vi "Write.vi"(8 "error in (no error)":errorcluster, 10 "write buffer":string, 11 "uCAN in":refnum<class "uCAN.lvclass">) -> (0 "error out":errorcluster)   [LabVIEW 2021, in "uCanDriver.lvlib" / "uCAN.lvclass"]
doc: "Writes given text on COM port"
uses:
  uCAN.lvclass
  uCAN.lvclass/uCAN.ctl
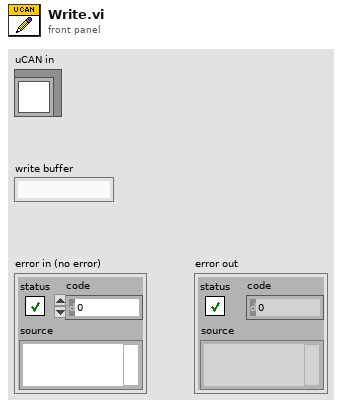
[diagram p1: front panel]
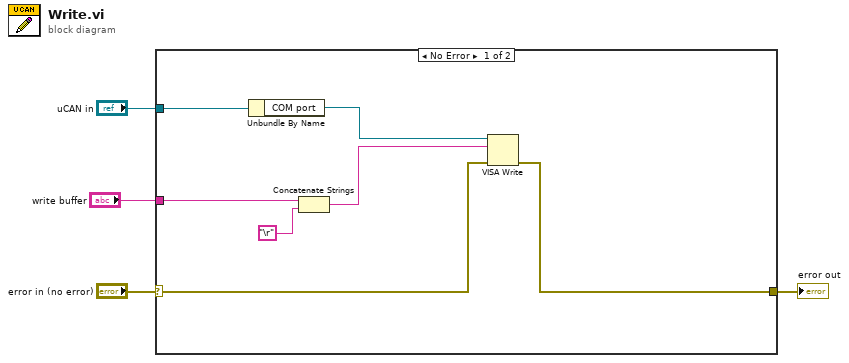
[diagram p0: block diagram]
diagram:
  n1 = case shown="No Error" "error in (no error)" {
    selector: "error in (no error)" -> [w9 w12]
    tunnel: [w8 w12] -> w3
    tunnel: "uCAN in" -> [w11 _]
    tunnel: "write buffer" -> [w7 _]
    frame No Error {
      n2 = Unbundle By Name(w11) -> ("COM port"=w10:refnum<visa-resource-name>)
      n3 = Concatenate Strings(w7, "\r") -> (w6:string)
      n4 = VISA Write(VISA resource name=w10, write buffer=w6, error in (no error)=w9) -> (error out=w8:errorcluster)  [unwired: 2 out]
    }
    frame Error {
    }
  }
  "error out" <- w3
